vi "Convert to Coordinates.vi"(8 "error in":errorcluster, 10 "Overlays":T1[](array[typedef]), 11 "BigMAQ in":refnum<class "BigMAQ.lvclass">) -> (0 "error out":errorcluster, 1 "Same Voltage":bool[](array[boolean]), 2 "Converted Overlays":T1[](array[typedef]), 3 "BigMAQ out":refnum<class "BigMAQ.lvclass">)   [LabVIEW 2019, in "BigMAQ.lvclass"]
uses:
  BigMAQ.lvclass
  Overlay.ctl
  BigMAQ.lvclass/BigMAQ.ctl
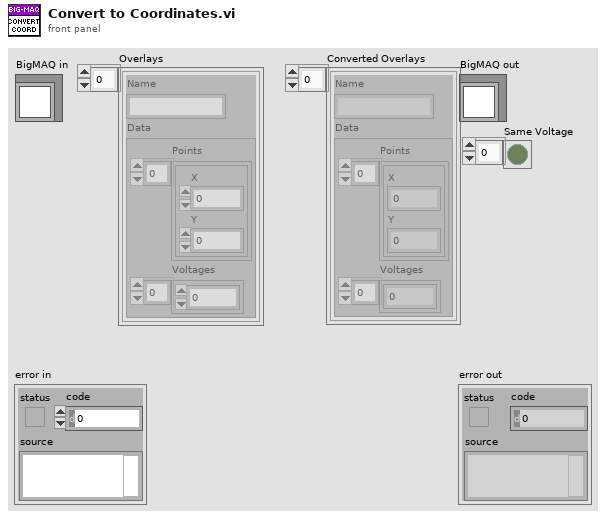
[diagram p1: front panel]
types:
  T1 = typedef "BigMAQ.lvclass/Overlay.ctl" = cluster{"Name":string, "Data":cluster{"Points":cluster{"X":dbl, "Y":dbl}[], "Voltages":dbl[]}}
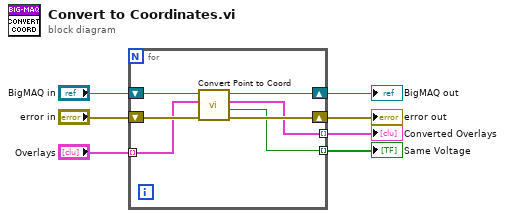
[diagram p0: block diagram]
diagram:
  n1 = for {
    tunnel: "Overlays" -> [w10] mode=indexing
    shift-right: [w13] -> w5
    shift-left: "BigMAQ in" -> [w14]
    shift-right: [w12] -> w4
    shift-left: "error in" -> [w11]
    tunnel: [w9] -> w3 mode=indexing
    tunnel: [w8] -> w2 mode=indexing
    n2 = call "Convert Point to Coord.vi"("error in"=w11, "Overlay"=w10, "BigMAQ in"=w14) -> ("error out"=w12:errorcluster, "Voltage Constant?"=w8:bool, "output cluster"=w9:T1, "BigMAQ out"=w13:refnum<class "BigMAQ.lvclass">)  [unwired: 5 in]
  }
  "error out" <- w4
  "BigMAQ out" <- w5
  "Converted Overlays" <- w3
  "Same Voltage" <- w2
